vi "总磷氨氮插入数据.vi"(0 "database":string, 1 "data":T2 {"单位" items=["ug/L", "mg/L", "ppm", "mg/m3", "cm", "ppb", "ug/m3", "%", "nmol/mol", "umol/mol", "MPN/L", "MPN/100ml", "ng/m3", "NTU", "无量纲", "ms/cm", "us/cm"]}, 3 "SN":string, 5 "table":string, 7 "测量模式":T1(ring)=enum."水样测试", 9 "数据标记表":string(combo)="N", 11 "error in (no error)":errorcluster) -> (15 "error out":errorcluster)   [LabVIEW 2016, in "斯坦道氨氮.lvlib"]
uses:
  <vilib>/Utility/sysdir.llb/System Directory Type.ctl
  <vilib>/addons/database/Connection.llb/DB Tools Open Connec (String).vi
  <vilib>/addons/database/Connection.llb/Conn Execute.vi
  <vilib>/addons/database/Recordset.llb/Rec Destroy - Connection.vi
  <vilib>/addons/database/Recordset.llb/Rec Fetch Recordset Data (R).vi
  <vilib>/addons/database/NI_Database_API.lvlib
panel:
  out "为空？":bool
  out "recordset data":variant[][](array[variant])
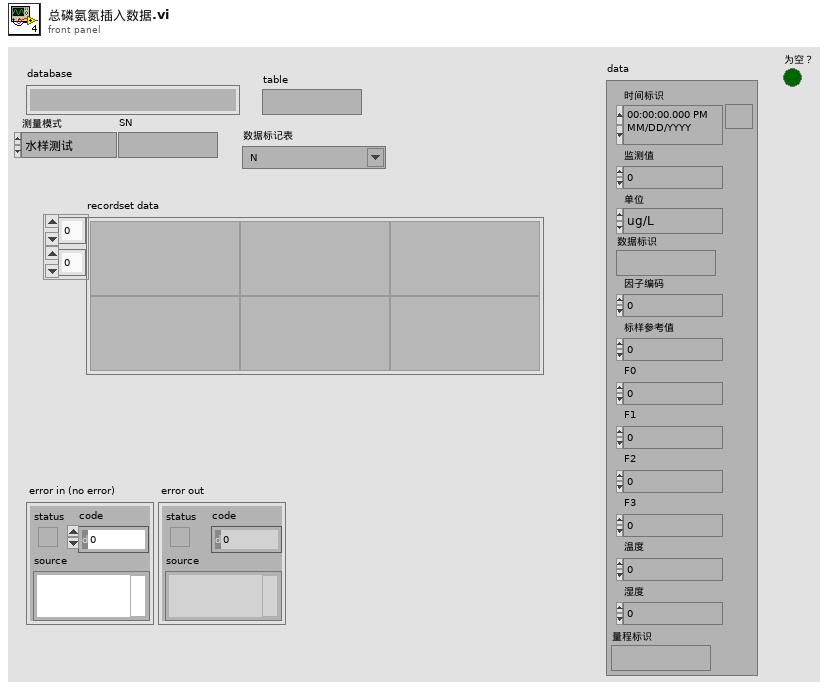
[diagram p1: front panel]
types:
  T1 = enum16{"维护数据", "水样测试", "标样核查", "零点核查", "跨度核查", "空白测试", "平行样测试", "加标回收", "空白校准", "标样校准", "初始化（清洗）"}
  T2 = cluster{"时间标识":timestamp, "监测值":sgl, "单位":u16, "数据标识":string, "因子编码":u32, "标样参考值":sgl, "F0":sgl, "F1":sgl, "F2":sgl, "F3":sgl, "温度":sgl, "湿度":sgl, "量程标识":string}
  T3 = typedef "System Directory Type.ctl" = i32
  T4 = typedef "NI_Database_API.lvlib/Conn ObjectReference.ctl" = refnum<k1>
  T5 = typedef "NI_Database_API.lvlib/Rec ObjectReference.ctl" = refnum<k1>
  T6 = cluster{"时间标识":timestamp, "测量模式":string, "数据类型":string, "监测值":sgl, "单位":string, "数据标识":string, "因子编码":string, "标样参考值":sgl, "F0":sgl, "F1":sgl, "F2":sgl, "F3":sgl, "温度":sgl, "湿度":sgl, "量程标识":string, "SN":string, "LastTime":timestamp}
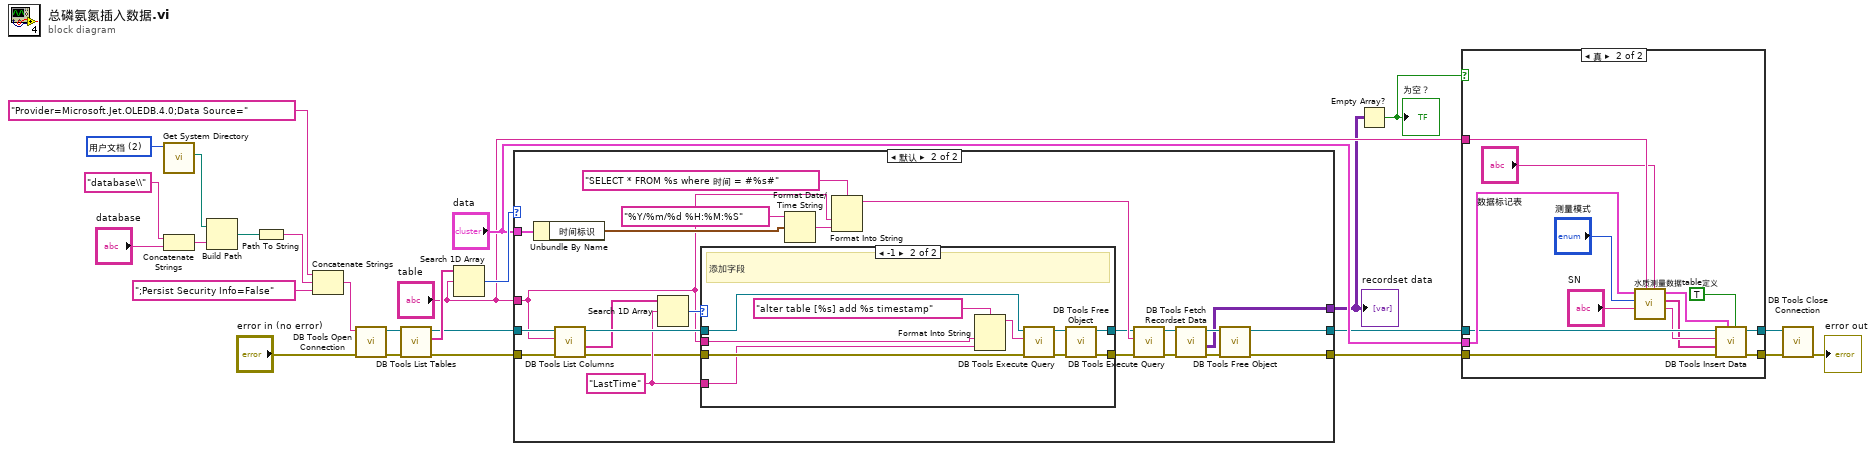
[diagram p0: block diagram]
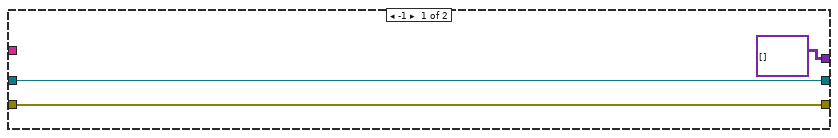
[diagram p2: hidden frame]
diagram:
  w25 = T3 2 items=["用户目录"=0, "用户桌面"=1, "用户文档"=2, "用户应用程序数据"=3, "用户设置"=4, "用户临时目录"=5, "公共文档"=6, "公共应用程序数据"=7, "公共设置"=8, "公共缓存"=13, "系统核心库"=9, "系统安装库"=10, "应用程序文件"=11, "启动盘根目录"=12] ("system directory type")
  n1 = call <vilib>:"Get System Directory.vi"("system directory type"=w25) -> ("system directory"=w23:path)  [unwired: 10 in]
  n2 = Concatenate Strings("database\\" ("condition"), "database") -> (w17:string)
  n3 = Build Path(base path=w23, name or relative path=w17) -> (appended path=w22:path)
  n4 = Path To String(path=w22) -> (string=w21:string)
  n5 = Concatenate Strings("Provider=Microsoft.Jet.OLEDB.4.0;Data Source=" ("condition"), w21, ";Persist Security Info=False" ("condition")) -> (w19:string)
  n6 = call-poly <vilib>:"DB Tools Open Connection.vi"("error in (no error)"="error in (no error)", "connection information"=w19) -> ("error out"=w15:errorcluster, "connection reference"=w16:T4)  [unwired: 6 in]
  n7 = call <vilib>:"DB Tools List Tables.vi"("error in (no error)"=w15, "connection reference"=w16) -> ("error out"=w4:errorcluster, "tables"=w14:string[], "connection reference out"=w5:T4)  [unwired: 3 in]
  n8 = Search 1D Array(1D array=w14, element="table") -> (index of element=w8:i32)  [unwired: 1 in]
  n9 = case shown="默认" w8 {
    tunnel: [variant[][] [] ("recordset data") w32] -> w3
    tunnel: [w29 w48] -> w2
    tunnel: [w28 w47] -> w1
    tunnel: w5 -> [w29 w34]
    tunnel: w4 -> [w28 w33]
    tunnel: "table" -> [_ w31]
    tunnel: "data" -> [_ w42]
    frame -1 {
    }
    frame Default {
      w40 = "LastTime" ("元素")
      n10 = Unbundle By Name(w42) -> ("时间标识"=w45:timestamp)
      n11 = call <vilib>:"DB Tools List Columns.vi"("error in (no error)"=w33, "table"=w31, "connection reference"=w34) -> ("error out"=w38:errorcluster, "columns"=w39:string[], "connection reference out"=w41:T4)  [unwired: 1 in, 1 out]
      n12 = Search 1D Array(1D array=w39, element=w40) -> (index of element=w37:i32)  [unwired: 1 in]
      n13 = case shown="-1" w37 {
        tunnel: w41 -> [w54 w62]
        tunnel: w38 -> [w53 w61]
        tunnel: w40 -> [_ w59]
        tunnel: [w54 w57] -> w36
        tunnel: [w53 w56] -> w35
        tunnel: w31 -> [_ w55]
        frame 0, Default {
        }
        frame -1 {
          # "添加字段"
          n14 = Format Into String(format string="alter table [%s] add %s timestamp", w55, w59) -> (resulting string=w58:string)  [unwired: 2 in, 1 out]
          n15 = call-poly <vilib>:"DB Tools Execute Query.vi"("error in (no error)"=w61, "SQL query"=w58, "connection reference"=w62) -> ("error out"=w63:errorcluster, "recordset reference"=w64:T5)  [unwired: 5 in]
          n16 = call-poly <vilib>:"DB Tools Free Object.vi"("error in (no error)"=w63, "recordset reference"=w64) -> ("error out"=w56:errorcluster, "connection reference"=w57:T4)  [unwired: 8 in]
        }
      }
      n17 = Format Date/Time String(time format string (%c)="%Y/%m/%d %H:%M:%S" ("时间格式字符串(%c)"), seconds (now)=w45) -> (date/time string=w43:string)  [unwired: 1 in]
      n18 = Format Into String(format string="SELECT * FROM %s where 时间 = #%s#" ("格式字符串"), w31, w43) -> (resulting string=w46:string)  [unwired: 2 in, 1 out]
      n19 = call-poly <vilib>:"DB Tools Execute Query.vi"("error in (no error)"=w35, "SQL query"=w46, "connection reference"=w36) -> ("error out"=w49:errorcluster, "recordset reference"=w52:T5)  [unwired: 5 in]
      n20 = call-poly <vilib>:"DB Tools Fetch Recordset Data.vi"("error in (no error)"=w49, "recordset reference"=w52) -> ("error out"=w50:errorcluster, "recordset data"=w32:variant[][], "recordset reference out"=w51:T5)  [unwired: 3 in]
      n21 = call-poly <vilib>:"DB Tools Free Object.vi"("error in (no error)"=w50, "recordset reference"=w51) -> ("error out"=w47:errorcluster, "connection reference"=w48:T4)  [unwired: 8 in]
    }
  }
  "recordset data" <- w3
  n22 = Empty Array?(array=w3) -> (empty?=w12:bool)
  "为空？" <- w12
  n23 = case shown="真" w12 {
    tunnel: "table" -> [_ w79]
    tunnel: "data" -> [_ w78]
    tunnel: w1 -> [w65 w76]
    tunnel: w2 -> [w66 w75]
    tunnel: [w66 w70] -> w11
    tunnel: [w65 w69] -> w10
    frame False {
    }
    frame True {
      n24 = call "水质测量数据table定义.vi"("数据标记表"="数据标记表", "table 输入"=w79, "SN"="SN", "测量模式"="测量模式", "data"=w78) -> ("table 输出"=w72:string, "columns"=w71:string[], "data输出"=w74:T6)  [unwired: 4 in]
      n25 = call <vilib>:"DB Tools Insert Data.vi"("create table? (F)"=TRUE, "data"=w74, "error in (no error)"=w76, "columns"=w71, "table"=w72, "connection reference"=w75) -> ("error out"=w69:errorcluster, "connection reference out"=w70:T4)  [unwired: 4 in]
    }
  }
  n26 = call <vilib>:"DB Tools Close Connection.vi"("error in (no error)"=w10, "connection reference"=w11) -> ("error out"=→"error out":errorcluster)  [unwired: 5 in]
